vi "Pressure Switch.vi"(6 "Puff time":u32, 8 "error in":errorcluster, 9 "Break In Time":u32, 10 "Pressure Box COM":refnum<visa-resource-name>, 11 "arduino pressure setting":T1) -> (0 "error out":errorcluster, 2 "Pressure Box COM out":refnum<visa-resource-name>)   [LabVIEW 2019]
uses:
  controls/arduino_pressure_setting.ctl
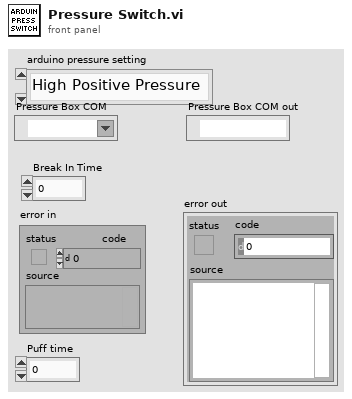
[diagram p1: front panel]
types:
  T1 = typedef "arduino_pressure_setting.ctl" = enum16{"High Positive Pressure", "Low Positive Pressure", "Atmospheric Pressure", "Low Vacuum", "High Vacuum", "Break In", "Puff"}
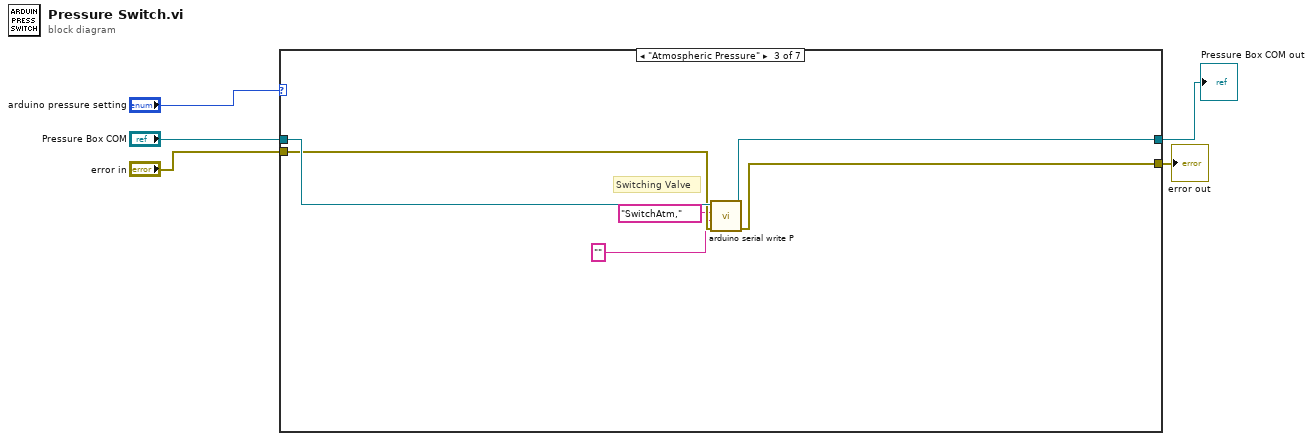
[diagram p0: block diagram]
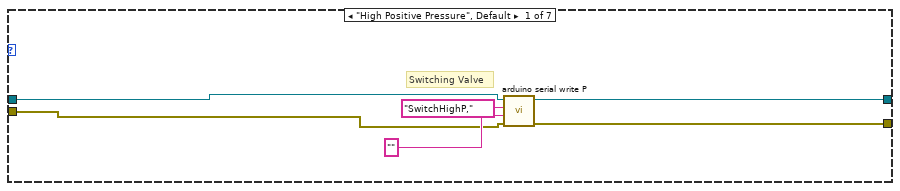
[diagram p2: hidden frame]
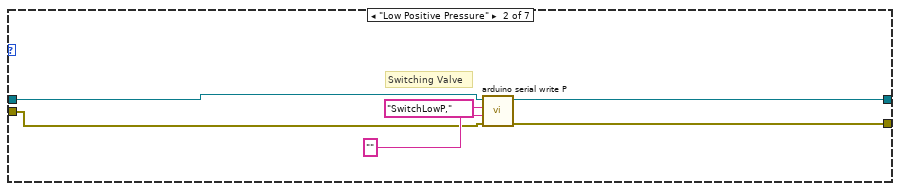
[diagram p3: hidden frame]
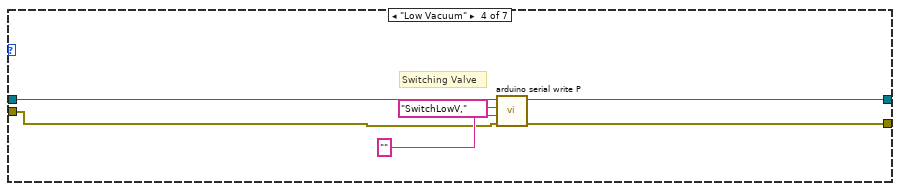
[diagram p4: hidden frame]
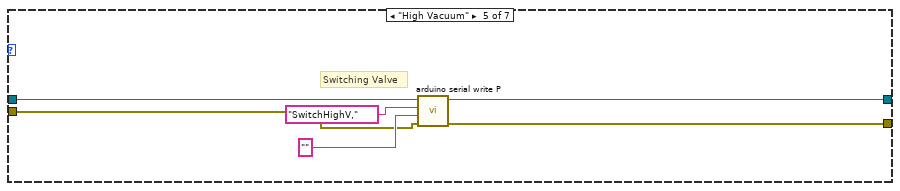
[diagram p5: hidden frame]
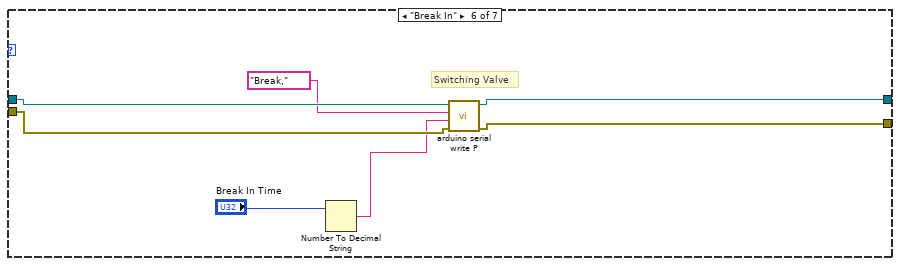
[diagram p6: hidden frame]
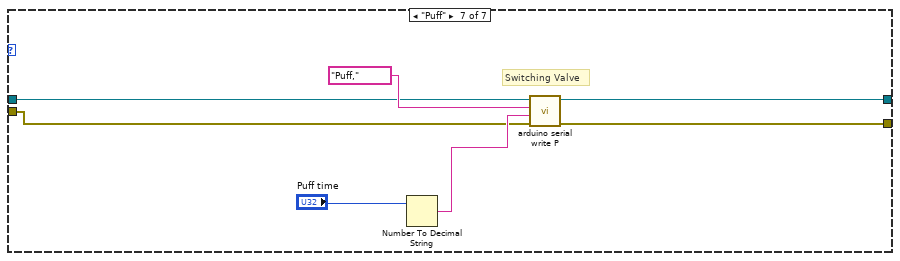
[diagram p7: hidden frame]
diagram:
  n1 = case shown="\"Atmospheric Pressure\"" "arduino pressure setting" {
    tunnel: "Pressure Box COM" -> [w9 w13 w23 w25 w31 w42 w46]
    tunnel: "error in" -> [w8 w12 w22 w24 w30 w41 w45]
    tunnel: [w7 w17 w18 w29 w35 w40 w43] -> w2
    tunnel: [w6 w16 w19 w28 w34 w39 w44] -> w1
    frame "High Positive Pressure", Default {
      # "Switching Valve"
      n2 = call "arduino serial write P.vi"("error in"=w8, "DAC value (0-1024)"="", "DAC output"="SwitchHighP,", "Pressure Box COM"=w9) -> ("error out"=w7:errorcluster, "Pressure Box COM out"=w6:refnum<visa-resource-name>)  [unwired: 6 in]
    }
    frame "Low Positive Pressure" {
      # "Switching Valve"
      n3 = call "arduino serial write P.vi"("error in"=w12, "DAC value (0-1024)"="", "DAC output"="SwitchLowP,", "Pressure Box COM"=w13) -> ("error out"=w17:errorcluster, "Pressure Box COM out"=w16:refnum<visa-resource-name>)  [unwired: 6 in]
    }
    frame "Atmospheric Pressure" {
      # "Switching Valve"
      n4 = call "arduino serial write P.vi"("error in"=w22, "DAC value (0-1024)"="", "DAC output"="SwitchAtm,", "Pressure Box COM"=w23) -> ("error out"=w18:errorcluster, "Pressure Box COM out"=w19:refnum<visa-resource-name>)  [unwired: 6 in]
    }
    frame "Low Vacuum" {
      # "Switching Valve"
      n5 = call "arduino serial write P.vi"("error in"=w24, "DAC value (0-1024)"="", "DAC output"="SwitchLowV,", "Pressure Box COM"=w25) -> ("error out"=w29:errorcluster, "Pressure Box COM out"=w28:refnum<visa-resource-name>)  [unwired: 6 in]
    }
    frame "High Vacuum" {
      # "Switching Valve"
      n6 = call "arduino serial write P.vi"("error in"=w30, "DAC value (0-1024)"="", "DAC output"="SwitchHighV,", "Pressure Box COM"=w31) -> ("error out"=w35:errorcluster, "Pressure Box COM out"=w34:refnum<visa-resource-name>)  [unwired: 6 in]
    }
    frame "Break In" {
      # "Switching Valve"
      n7 = Number To Decimal String(number="Break In Time") -> (decimal integer string=w36:string)  [unwired: 1 in]
      n8 = call "arduino serial write P.vi"("error in"=w41, "DAC value (0-1024)"=w36, "DAC output"="Break,", "Pressure Box COM"=w42) -> ("error out"=w40:errorcluster, "Pressure Box COM out"=w39:refnum<visa-resource-name>)  [unwired: 6 in]
    }
    frame "Puff" {
      # "Switching Valve"
      n9 = Number To Decimal String(number="Puff time") -> (decimal integer string=w47:string)  [unwired: 1 in]
      n10 = call "arduino serial write P.vi"("error in"=w45, "DAC value (0-1024)"=w47, "DAC output"="Puff,", "Pressure Box COM"=w46) -> ("error out"=w43:errorcluster, "Pressure Box COM out"=w44:refnum<visa-resource-name>)  [unwired: 6 in]
    }
  }
  "error out" <- w2
  "Pressure Box COM out" <- w1
